vi "Get_values.vi"(1 "DAC values":sgl[][](array[numeric]), 2 "Inst_array":T2(array[cluster]), 3 "Temp file path":path) -> (0 "Initial positions":T1(array[cluster]))   [LabVIEW 2013]
uses:
  <vilib>/addons/h5labview2/file/H5Fmode.ctl
  <vilib>/addons/h5labview2/base/lib_path.vi
  <vilib>/addons/h5labview2/base/H5Equery.vi
  <vilib>/addons/h5labview2/dataset/H5Dwrite.llb/H5Dwrite.xnode
  <vilib>/addons/h5labview2/file/H5F.lvlib
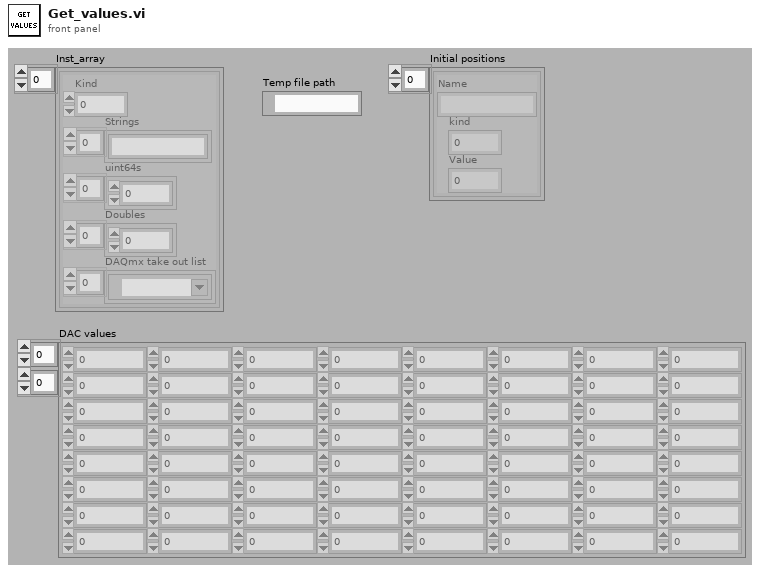
[diagram p1: front panel]
types:
  T1 = cluster{"Name":string, "kind":u64, "Value":dbl}[]
  T2 = cluster{"Kind":u16, "Strings":string[], "uint64s":u64[], "Doubles":dbl[], "DAQmx take out list":refnum<k21>[]}[]
  T3 = typedef "H5F.lvlib/H5Fmode.ctl" = enum16{"read-only", "read-write", "overwrite", "create new", "open or create"}
  T4 = cluster{string, "Kind":u16, "DAC value (sgl)":sgl}
  T5 = typedef "hid_t.ctl" = i32
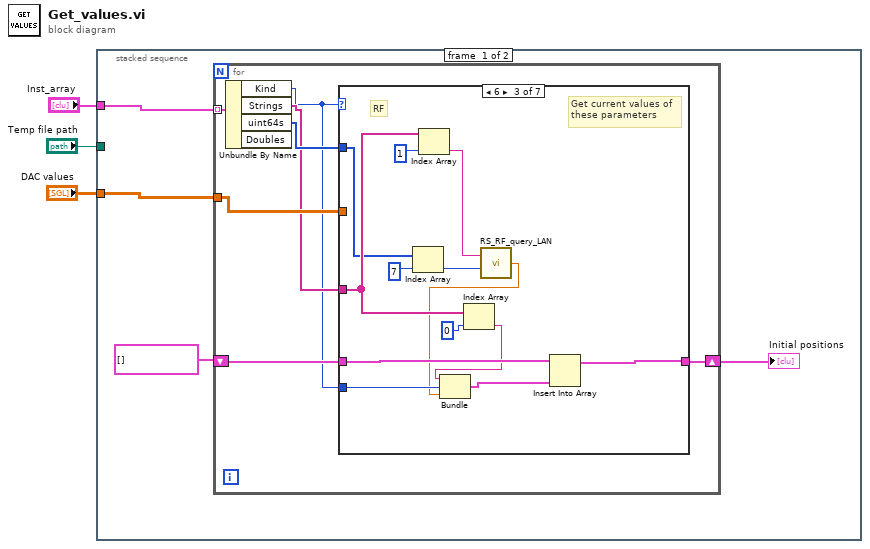
[diagram p0: block diagram]
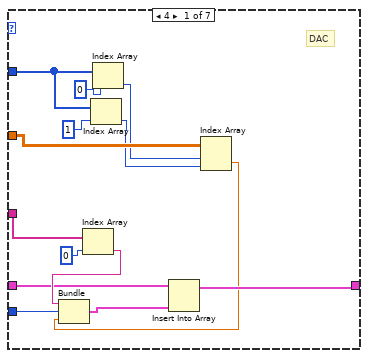
[diagram p2: hidden frame]
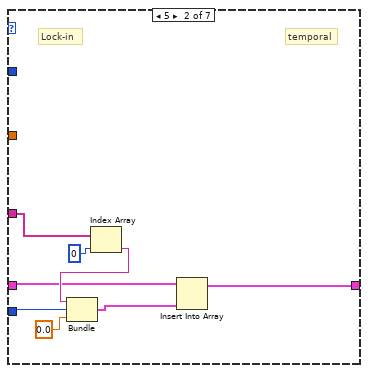
[diagram p3: hidden frame]
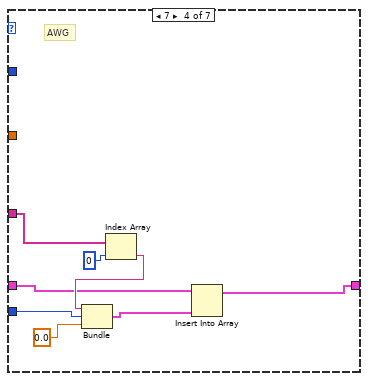
[diagram p4: hidden frame]
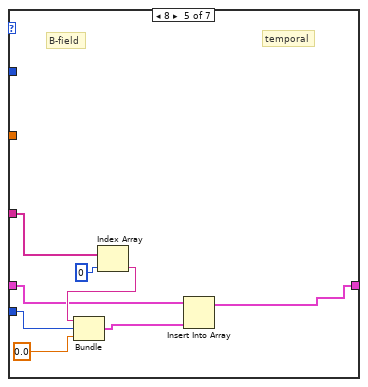
[diagram p5: hidden frame]
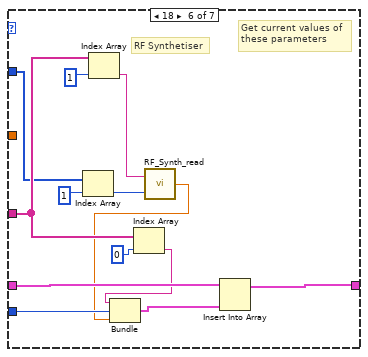
[diagram p6: hidden frame]
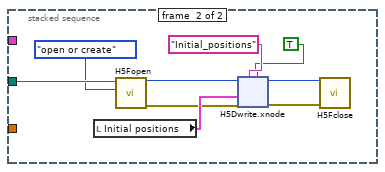
[diagram p8: hidden frame]
diagram:
  n1 = stacked-sequence {
    tunnel: "DAC values" -> [w7 _]
    tunnel: "Inst_array" -> [w6 _]
    tunnel: "Temp file path" -> [_ w85]
    frame #0 {
      n2 = for {
        tunnel: w6 -> [w14] mode=indexing
        tunnel: w7 -> [w11]
        shift-right: [w12] -> w4
        shift-left: T1 [] ("Initial move") -> [w13]
        n3 = Unbundle By Name(w14) -> ("Kind"=w8:u16, "Strings"=w9:string[], "uint64s"=w10:u64[])  [unwired: 1 out]
        n4 = case shown="6" w8 {
          tunnel: [w17 w34 w44 w53 w61 w74 w79] -> w12
          tunnel: w13 -> [w18 w33 w49 w54 w62 w78 w79]
          tunnel: w11 -> [w28 _ _ _ _ _ _]
          tunnel: w10 -> [w27 _ w38 _ _ w69 _]
          tunnel: w9 -> [w21 w32 w47 w55 w63 w76 _]
          tunnel: w8 -> [w19 w31 w48 w52 w60 w77 _]
          frame 4 {
            # "DAC"
            n5 = Index Array(array=w21, index=0) -> (element=w20:string)
            n6 = Index Array(array=w27, index=1) -> (element=w23:u64)
            n7 = Index Array(array=w27, index=0) -> (element=w24:u64)
            n8 = Index Array(array=w28, index (row)=w24, index (col)=w23) -> (element=w16:sgl)
            n9 = Bundle(w20, "Kind"=w19, "DAC value (sgl)"=w16) -> (w15:T4)  [unwired: 1 in]
            n10 = Insert Into Array(array=w18, new element=w15) -> (w17:T1)  [unwired: 1 in]
          }
          frame 5 {
            # "temporal"
            # "Lock-in"
            n11 = Index Array(array=w32, index=0) -> (element=w35:string)
            n12 = Bundle(w35, "Kind"=w31, 0.0) -> (w29:cluster{string, "Kind":u16, dbl})  [unwired: 1 in]
            n13 = Insert Into Array(array=w33, new element=w29) -> (w34:T1)  [unwired: 1 in]
          }
          frame 6 {
            # "Get current values of\nthese parameters"
            # "RF"
            n14 = Index Array(array=w38, index=7) -> (element=w37:u64)
            n15 = Index Array(array=w47, index=1) -> (element=w45:string)
            n16 = Index Array(array=w47, index=0) -> (element=w40:string)
            n17 = call "RS_RF_query_LAN.vi"("Parameter"=w37, "IP address"=w45) -> ("value"=w42:dbl)
            n18 = Bundle(w40, "Kind"=w48, "value"=w42) -> (w41:cluster{string, "Kind":u16, "value":dbl})  [unwired: 1 in]
            n19 = Insert Into Array(array=w49, new element=w41) -> (w44:T1)  [unwired: 1 in]
          }
          frame 7 {
            # "AWG"
            n20 = Index Array(array=w55, index=0) -> (element=w56:string)
            n21 = Bundle(w56, "Kind"=w52, 0.0) -> (w50:cluster{string, "Kind":u16, dbl})  [unwired: 1 in]
            n22 = Insert Into Array(array=w54, new element=w50) -> (w53:T1)  [unwired: 1 in]
          }
          frame 8 {
            # "temporal"
            # "B-field"
            n23 = Index Array(array=w63, index=0) -> (element=w64:string)
            n24 = Bundle(w64, "Kind"=w60, 0.0) -> (w58:cluster{string, "Kind":u16, dbl})  [unwired: 1 in]
            n25 = Insert Into Array(array=w62, new element=w58) -> (w61:T1)  [unwired: 1 in]
          }
          frame 18 {
            # "RF Synthetiser"
            # "Get current values of\nthese parameters"
            n26 = Index Array(array=w69, index=1) -> (element=w67:u64)
            n27 = Index Array(array=w76, index=1) -> (element=w68:string)
            n28 = Index Array(array=w76, index=0) -> (element=w71:string)
            n29 = call "RF_Synth_read.vi"("Parameter"=w67, "Address"=w68) -> ("Value"=w66:dbl)
            n30 = Bundle(w71, "Kind"=w77, "Value"=w66) -> (w72:cluster{string, "Kind":u16, "Value":dbl})  [unwired: 1 in]
            n31 = Insert Into Array(array=w78, new element=w72) -> (w74:T1)  [unwired: 1 in]
          }
          frame 100, Default {
          }
        }
      }
      "Initial positions" <- w4
    }
    frame #1 {
      n32 = local read "Initial positions"() -> (w86:T1)
      n33 = call <vilib>:"H5Fopen.vi"("mode (read-only)"=H5Fmode."open or create" ("mode"), "path"=w85) -> ("error out"=w82:errorcluster, "ref out"=w83:T5)  [unwired: 8 in]
      n34 = xnode "H5Dwrite.xnode"("replace? (F)"=TRUE, "dataset name"="Initial_positions", "error in (no error)"=w82, "data"=w86, "ref in"=w83) -> ("error out"=w80:errorcluster, "ref out"=w81:i32)  [unwired: 2 in, 1 out]
      n35 = call <vilib>:"H5Fclose.vi"("error in (no error)"=w80, "ref"=w81) -> ()  [unwired: 9 in, 1 out]
    }
  }
